vi "Increment Build Number.vi"(0 "NI Build Specification in":refnum<class "NIPKG_LV.lvclass">, 11 "error in (no error)":errorcluster) -> (4 "NI Build Specification out":refnum<class "NIPKG_LV.lvclass">, 15 "error out":errorcluster)   [LabVIEW 2017, in "CL_G3_VIComponentBuilder.lvlib" / "NIPKG_LV.lvclass"]
doc: "Upgrades the version number of the NI Package in the LabVIEW project build spec."
uses:
  NIPKG_LV.lvclass
  C:/Tool Chain Support/Software Module Builder/Source/Exports/NI Build Specification_LV/NI Build Specification_LV.lvclass
  C:/Tool Chain Support/Software Module Builder/Source/Exports/Exports/Export.lvclass
  NI Build Specification_LV/NI Build Specification_LV.lvclass/NI Build Specification_LV.ctl
  Exports/Export.lvclass/Export.ctl
  NI Build Specification_LV/Accessors/Read Build Number XML Prop Name.vi
  Exports/Accessors/Read Exported Build Specification Path.vi
  NI Build Specification_LV/NI Build Specification_LV.lvclass
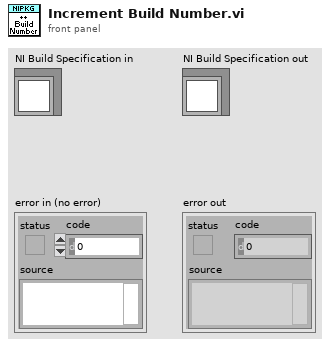
[diagram p1: front panel]
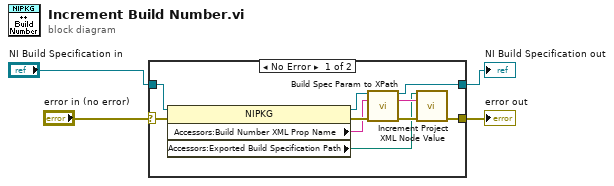
[diagram p0: block diagram]
diagram:
  n1 = case shown="No Error" "error in (no error)" {
    selector: "error in (no error)" -> [w13 w15]
    tunnel: "NI Build Specification in" -> [w14 w16]
    tunnel: [w7 w16] -> w3
    tunnel: [w12 w15] -> w2
    frame No Error {
      n2 = property class="NIPKG"(reference=w14, error in=w13) -> (reference out=w11:refnum<class "NIPKG_LV.lvclass">, error out=w9:errorcluster, "Accessors:Build Number XML Prop Name"=w8:string, "Accessors:Exported Build Specification Path"=w5:path)
      n3 = call-dynamic "Build Spec Param to XPath.vi"("NI Build Specification"=w11, "Build Spec Parameter Name"=w8, "error in (no error)"=w9) -> ("NI Build Specification"=w7:refnum<class "NIPKG_LV.lvclass">, "XPath to the specific build Spec Property"=w10:string, "error out"=w6:errorcluster)  [unwired: 10 in]
      n4 = call "Increment Project XML Node Value.vi"("path to XML document"=w5, "Xpath to Node"=w10, "error in (no error)"=w6) -> ("error out"=w12:errorcluster)  [unwired: 12 in]
    }
    frame Error {
    }
  }
  "error out" <- w2
  "NI Build Specification out" <- w3
